vi "Save_Scan_macro.vi"(8 "error in (no error)":errorcluster, 10 "Paths":T1, 11 "Application":refnum<k7>) -> (0 "error out":errorcluster, 3 "BMP":picture)   [LabVIEW 2016]
uses:
  Type-Defs/Paths.ctl
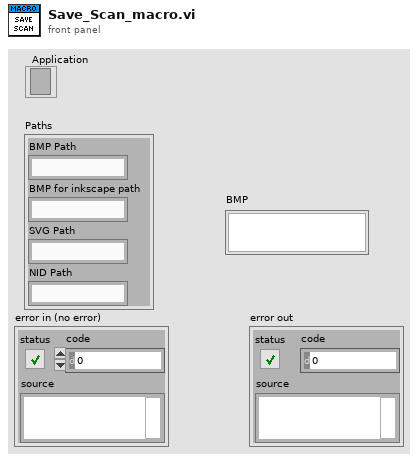
[diagram p1: front panel]
types:
  T1 = typedef "Paths.ctl" = cluster{"BMP Path":string, "BMP for inkscape path":string, "SVG Path":string, "NID Path":string}
  T2 = cluster{"CenterPosX":dbl, "CenterPosY":dbl, "ImageHeight":dbl, "ImageWidth":dbl}
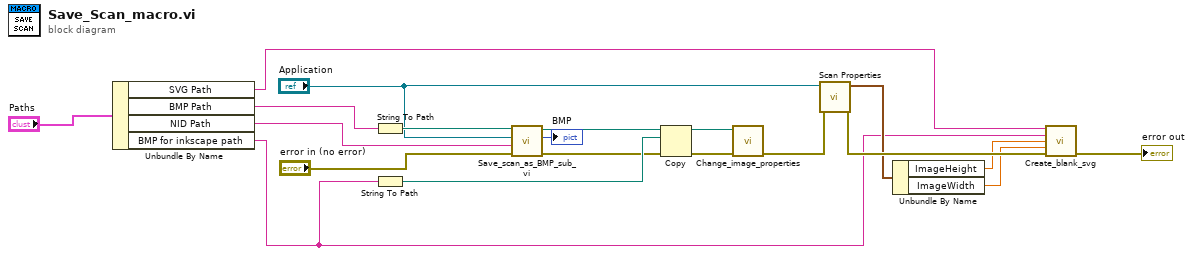
[diagram p0: block diagram]
diagram:
  n1 = Unbundle By Name("Paths") -> ("SVG Path"=w1:string, "BMP Path"=w4:string, "NID Path"=w3:string, "BMP for inkscape path"=w2:string)
  n2 = String To Path(string=w4) -> (path=w19:path)
  n3 = String To Path(string=w2) -> (path=w17:path)
  n4 = call "Save_scan_as_BMP_sub_vi.vi"("error in (no error)"="error in (no error)", "NID Path In"=w3, "Application"="Application", "BMP Path In"=w19) -> ("Error Out"=w16:errorcluster, "BMP"=→"BMP":picture, "BMP Path Out"=w20:path)  [unwired: 5 in]
  n5 = Copy(8:w16, 10:w17, 11:w20) -> (0:w15:errorcluster, 3:w18:path)  [unwired: 2 in, 1 out]
  n6 = call "Change_image_properties.vi"("error in (no error)"=w15, "Path In"=w18) -> ("error out"=w14:errorcluster)  [unwired: 8 in, 1 out]
  n7 = call "Scan Properties.vi"("error in (no error)"=w14, "Application"="Application") -> ("error out"=w13:errorcluster, "Scan Properties"=w12:T2)  [unwired: 8 in]
  n8 = Unbundle By Name(w12) -> ("ImageHeight"=w11:dbl, "ImageWidth"=w10:dbl)
  n9 = call "Create_blank_svg.vi"("SVG Path"=w1, "BMP for inkscape path"=w2, "HEIGHT"=w11, "WIDTH"=w10, "error in"=w13) -> ("error out"=→"error out":errorcluster)  [unwired: 9 in, 1 out]
